vi "SCM Signal Conditioner.vi"(4 "Signals":waveform(dbl)[](array[waveform])) -> (1 "Conditioned Signals":waveform(dbl)[](array[waveform]))   [LabVIEW 2013, in "Breakdown Acoustics Controls.lvlib"]
uses:
  Breakdown Acoustics Controls/Breakdown Acoustics Controls.lvlib
  <vilib>/Analysis/2dsp.llb/Real FFT.vi
  <vilib>/measure/maresamp.llb/Resample Waveform (single shot).vi
  <vilib>/measure/NI_MAPro.lvlib
  <vilib>/Analysis/NI_AALPro.lvlib
panel:
  out "Input Signals":waveform(dbl)[](graph)
  out "Conditioned Signal":waveform(dbl)[](graph)
  out "FFT Imag":dbl[][](graph)
  out "FFT Real":dbl[][](graph)
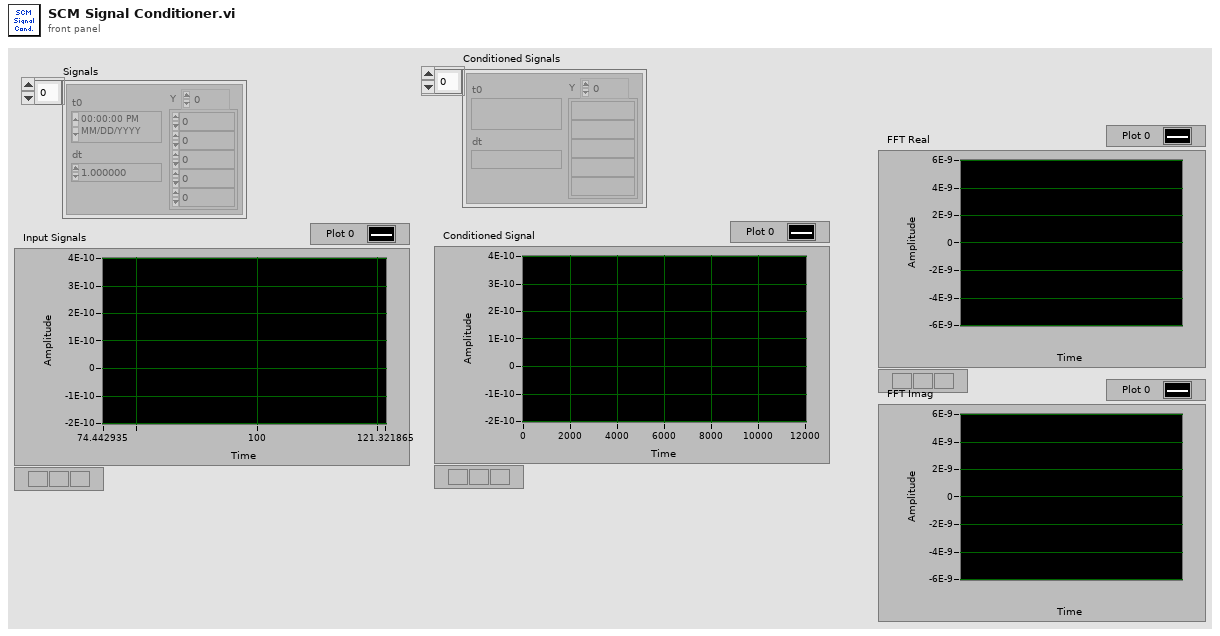
[diagram p1: front panel]
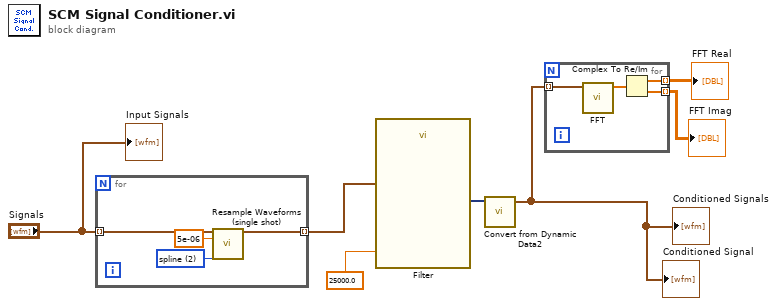
[diagram p0: block diagram]
diagram:
  n1 = for {
    tunnel: "Signals" -> [w8] mode=indexing
    tunnel: [w11] -> w7 mode=indexing
    w9 = u16 2 items=["coerce", "linear", "spline", "FIR filter"] ("interpolation mode")
    n2 = call-poly <vilib>:"Resample Waveforms (single shot).vi"("waveform in"=w8, "dt"=5e-06, "interpolation mode"=w9) -> ("resampled waveform out"=w11:waveform(dbl))  [unwired: 9 in, 3 out]
  }
  n3 = call "Filter"("Lower Cut-Off"=25000.0, "Signal"=w7) -> ("Filtered Signal"=w2:dynamicdata)  [unwired: 8 in, 1 out]
  n4 = call "Convert from Dynamic Data2"("Dynamic Data Type"=w2) -> ("Array of Waveform"=w1:waveform(dbl)[])  [unwired: 3 in]
  "Conditioned Signal" <- w1
  "Conditioned Signals" <- w1
  n5 = for {
    tunnel: w1 -> [w13] mode=indexing
    tunnel: [w15] -> w5 mode=indexing
    tunnel: [w14] -> w4 mode=indexing
    n6 = call-poly <vilib>:"FFT.vi"("X"=w13) -> ("FFT {X}"=w12:cdb[])  [unwired: 9 in, 1 out]
    n7 = Complex To Re/Im(x + iy=w12) -> (x=w15:dbl[], y=w14:dbl[])
  }
  "FFT Real" <- w5
  "FFT Imag" <- w4
  "Input Signals" <- "Signals"
